vi "test Call Mock Transceiver Interface.vi"(8 "error in (no error)":errorcluster, 11 "TestCase in":refnum<class "Transceiver Test Cases.lvclass">) -> (0 "error out":errorcluster, 3 "TestCase out":refnum<class "Transceiver Test Cases.lvclass">)   [LabVIEW 2017, in "Transceiver Test Cases.lvclass"]
uses:
  Transceiver Test Cases.lvclass
  Configuration/Public/Controls/DSF Engine Transfer Group Configuration.ctl
  Configuration/Public/Controls/DSF Direction.ctl
  Configuration/Public/Controls/DSF Timing Info.ctl
  Configuration/Public/Controls/DSF Engine Transfer Configuration.ctl
  Configuration/Public/Controls/DSF Byte Order.ctl
  Configuration/Public/Controls/DSF Engine Channel Configuration.ctl
  Configuration/Public/Controls/DSF Data Type.ctl
  Configuration/Public/Controls/DSF Settings Info.ctl
  MockTransceiver.lvclass
  Engine/Classes/Transfer Group/Transfer Group.lvclass
  <vilib>/addons/_JKI Toolkits/VI Tester/TestCase.llb/TestCase.lvclass
  DSF Core.lvlib
  C:/Program Files (x86)/National Instruments/LabVIEW 2017/vi.lib/addons/_JKI Toolkits/VI Tester/TestCase.llb/TestCase.lvclass
panel:
  out "# elements after receive":i32
  out "# elements after transmit":i32
  out "Queue was destroyed?":bool
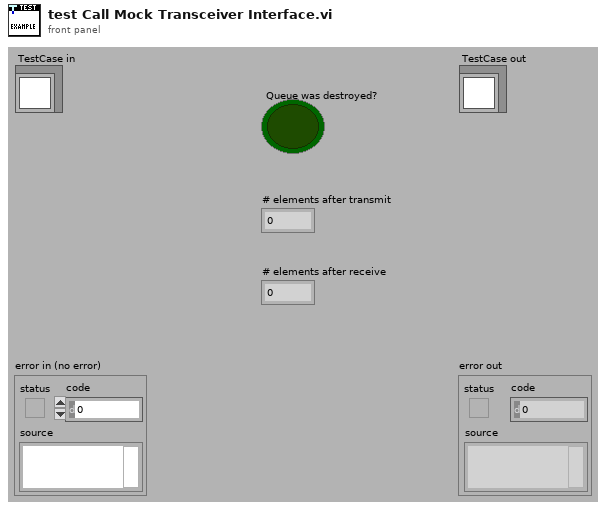
[diagram p1: front panel]
types:
  T1 = typedef "DSF Core.lvlib/DSF Settings Info.ctl" = cluster{"key":string, "value":string}[]
  T2 = typedef "DSF Core.lvlib/DSF Engine Transfer Group Configuration.ctl" = cluster{"name":string, "direction":T3, "cycle timing":T4, "Transfers":T5[], "settings":T1}
  T3 = typedef "DSF Core.lvlib/DSF Direction.ctl" = enum8{"Tx", "Rx"}
  T4 = typedef "DSF Core.lvlib/DSF Timing Info.ctl" = cluster{"priority":u64, "decimation":u64, "offset":u64}
  T5 = typedef "DSF Core.lvlib/DSF Engine Transfer Configuration.ctl" = cluster{"name":string, "byte order":T6, "channel configurations":T7[], "settings":T1}
  T6 = typedef "DSF Core.lvlib/DSF Byte Order.ctl" = enum8{"big-endian", "little-endian"}
  T7 = typedef "DSF Core.lvlib/DSF Engine Channel Configuration.ctl" = cluster{"engine offset":u64, "name":string, "data type":T8, "count":u64, "buffer offset":u64}
  T8 = typedef "DSF Core.lvlib/DSF Data Type.ctl" = enum8{"Bool", "SGL", "DBL", "I8", "I16", "I32", "I64", "U8", "U16", "U32", "U64"}
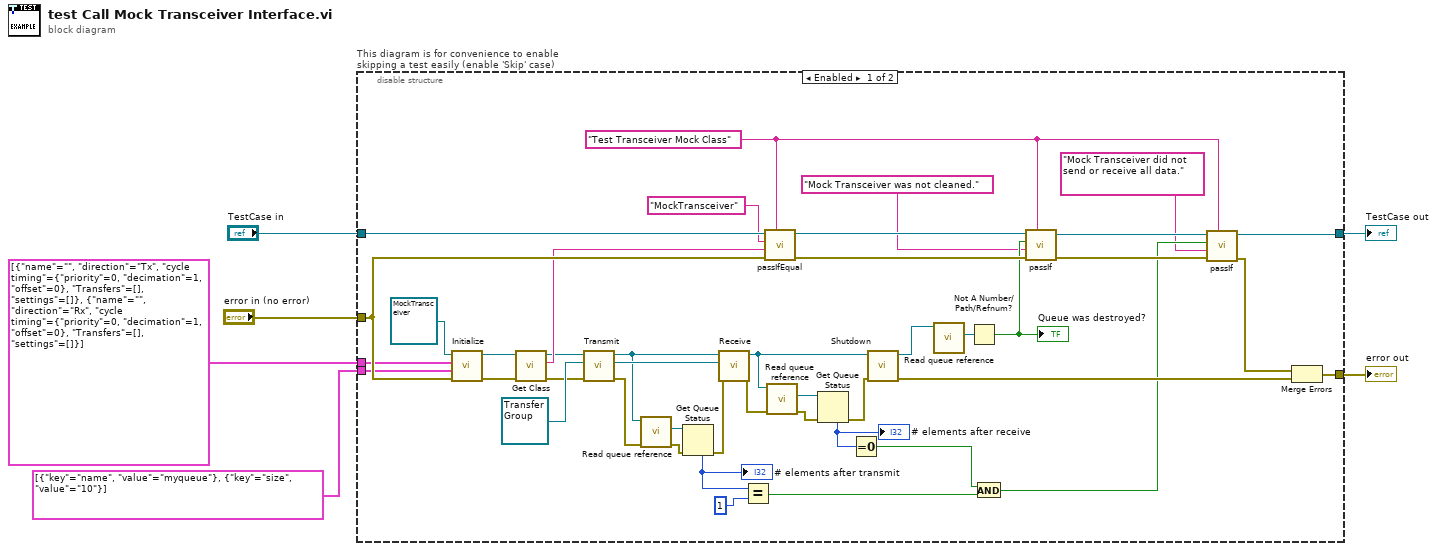
[diagram p0: block diagram]
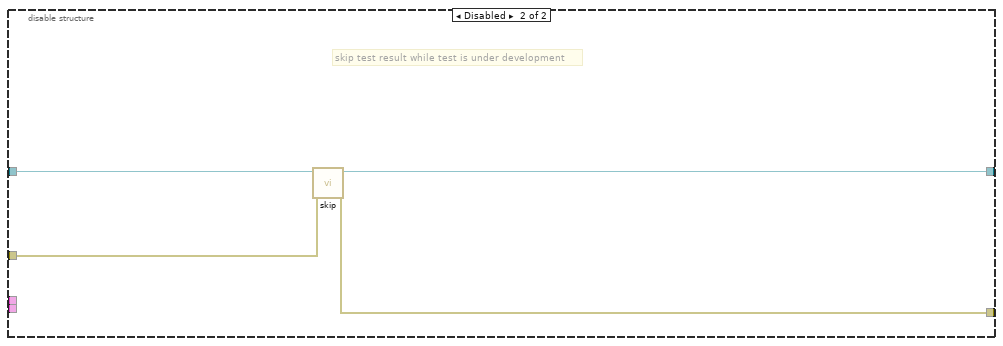
[diagram p2: hidden frame]
diagram:
  n1 = disable-structure "This diagram is for convenience to enable skipping a test easily (enable 'Skip' case)" shown="Enabled" {
    disable-tunnel: "TestCase in" -> [w49 w53]
    disable-tunnel: [w19 w51] -> w3
    disable-tunnel: [w48 w52] -> w5
    disable-tunnel: "error in (no error)" -> [w46 w50]
    disable-tunnel: T2[] [{"name"="", "direction"=enum."Tx", "cycle timing"={"priority"=0, "decimation"=1, "offset"=0}, "Transfers"=[], "settings"=[]}, {"name"="", "direction"=enum."Rx", "cycle timing"={"priority"=0, "decimation"=1, "offset"=0}, "Transfers"=[], "settings"=[]}] ("Transfer Groups Configurations") -> [w39 _]
    disable-tunnel: T1 [{"key"="name", "value"="myqueue"}, {"key"="size", "value"="10"}] ("transceiver settings") -> [w29 _]
    frame Enabled {
      w20 = "Test Transceiver Mock Class" ("custom report message (\"\")")
      n2 = call-dynamic "Initialize.vi"("error in (no error)"=w46, "transceiver settings"=w29, "Transfer Groups Configurations"=w39, "MockTransceiver in"=refnum<class "MockTransceiver.lvclass"> refnum) -> ("error out"=w30:errorcluster, "MockTransceiver out"=w31:refnum<class "MockTransceiver.lvclass">)  [unwired: 6 in]
      n3 = call-dynamic "Get Class.vi"("error in (no error)"=w30, "MockTransceiver in"=w31) -> ("error out"=w32:errorcluster, "class"=w44:string, "MockTransceiver out"=w33:refnum<class "MockTransceiver.lvclass">)  [unwired: 7 in]
      n4 = call-dynamic "Transmit.vi"("error in (no error)"=w32, "Transfer Group in"=refnum<class "Transfer Group.lvclass"> refnum, "MockTransceiver in"=w33) -> ("error out"=w27:errorcluster, "Transfer Group out"=w34:refnum<class "Transfer Group.lvclass">, "MockTransceiver out"=w28:refnum<class "MockTransceiver.lvclass">)  [unwired: 6 in]
      n5 = call-dynamic "Read queue reference.vi"("error in (no error)"=w27, "MockTransceiver in"=w28) -> ("error out"=w16:errorcluster, "queue reference"=w26:refnum<queue>)  [unwired: 7 in, 1 out]
      n6 = Get Queue Status(queue=w26, error in (no error)=w16) -> (error out=w15:errorcluster, # elements in queue=w23:i32)  [unwired: 1 in, 6 out]
      "# elements after transmit" <- w23
      n7 = call-dynamic "Receive.vi"("error in (no error)"=w15, "Transfer Group in"=w34, "MockTransceiver in"=w28) -> ("error out"=w17:errorcluster, "MockTransceiver out"=w12:refnum<class "MockTransceiver.lvclass">)  [unwired: 6 in, 1 out]
      n8 = Equal?(x=w23, y=1) -> (x = y?=w9:bool)
      n9 = call-dynamic "passIfEqual.vi"("custom report message (\"\")"=w20, "error in (no error)"=w46, "y"=w44, "x"="MockTransceiver", "TestCase in"=w49) -> ("error out"=w42:errorcluster, "TestCase out"=w43:refnum<class "Transceiver Test Cases.lvclass">)  [unwired: 5 in]
      n10 = call-dynamic "Read queue reference.vi"("error in (no error)"=w17, "MockTransceiver in"=w12) -> ("error out"=w14:errorcluster, "queue reference"=w11:refnum<queue>)  [unwired: 7 in, 1 out]
      n11 = Get Queue Status(queue=w11, error in (no error)=w14) -> (error out=w13:errorcluster, # elements in queue=w21:i32)  [unwired: 1 in, 6 out]
      "# elements after receive" <- w21
      n12 = Equal To 0?(x=w21) -> (x = 0?=w10:bool)
      n13 = call-dynamic "Shutdown.vi"("error in (no error)"=w13, "MockTransceiver in"=w12) -> ("error out"=w45:errorcluster, "MockTransceiver out"=w37:refnum<class "MockTransceiver.lvclass">)  [unwired: 8 in]
      n14 = call-dynamic "Read queue reference.vi"("MockTransceiver in"=w37) -> ("queue reference"=w38:refnum<queue>)  [unwired: 8 in, 2 out]
      n15 = Not A Number/Path/Refnum?(number/path/refnum=w38) -> (NaN/Path/Refnum?=w41:bool)
      "Queue was destroyed?" <- w41
      n16 = And(x=w10, y=w9) -> (x .and. y?=w8:bool)
      n17 = call-dynamic "passIf.vi"("custom report message (\"\")"=w20, "error in (no error)"=w42, "message (\"\")"="Mock Transceiver was not cleaned." ("message (\"\")"), "pass"=w41, "TestCase in"=w43) -> ("error out"=w25:errorcluster, "TestCase out"=w24:refnum<class "Transceiver Test Cases.lvclass">)  [unwired: 5 in]
      n18 = call-dynamic "passIf.vi"("custom report message (\"\")"=w20, "error in (no error)"=w25, "message (\"\")"="Mock Transceiver did not send or receive all data." ("message (\"\")"), "pass"=w8, "TestCase in"=w24) -> ("error out"=w18:errorcluster, "TestCase out"=w19:refnum<class "Transceiver Test Cases.lvclass">)  [unwired: 5 in]
      n19 = Merge Errors(w18, w45) -> (w48:errorcluster)
    }
    frame Disabled {
      # "skip test result while test is under development"
      n20 = call <vilib>:"skip.vi"("error in (no error)"=w50, "TestCase in"=w53) -> ("error out"=w52:errorcluster, "TestCase out"=w51:refnum<class "Transceiver Test Cases.lvclass">)  [unwired: 8 in]
    }
  }
  "error out" <- w5
  "TestCase out" <- w3
